vi "Convert to MessagePackT format byte.vi"(8 "error in (no error)":errorcluster, 11 "Object type":T1) -> (0 "error out":errorcluster, 3 "Byte":u8)   [LabVIEW 2020]
uses:
  MsgPack Object Types.ctl
  <vilib>/ErrorRing/Error Ring.xnode
  MessagePack.lvclass/MessagePack.ctl
  MessagePack.lvclass
  <vilib>/Utility/error.llb/Error Cluster From Error Code.vi
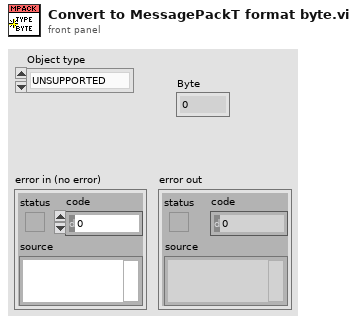
[diagram p1: front panel]
types:
  T1 = typedef "MessagePack.lvlib/MessagePack.lvclass/MsgPack Object Types.ctl" = enum16{"UNSUPPORTED", "POSINT", "NEGINT", "FIXMAP", "FIXARRAY", "FIXSTR", "NIL", "FALSE", "TRUE", "BIN8", "BIN16", "BIN32", "EXT8", "EXT16", "EXT32", "FLOAT32", "FLOAT64", "UINT8", "UINT16", "UINT32", "UINT64", "INT8", "INT16", "INT32", "INT64", "FIXEXT1", "FIXEXT2", "FIXEXT4", "FIXEXT8", "FIXEXT16", "STR8", "STR16", "STR32", "ARRAY16", "ARRAY32", "MAP16", "MAP32"}
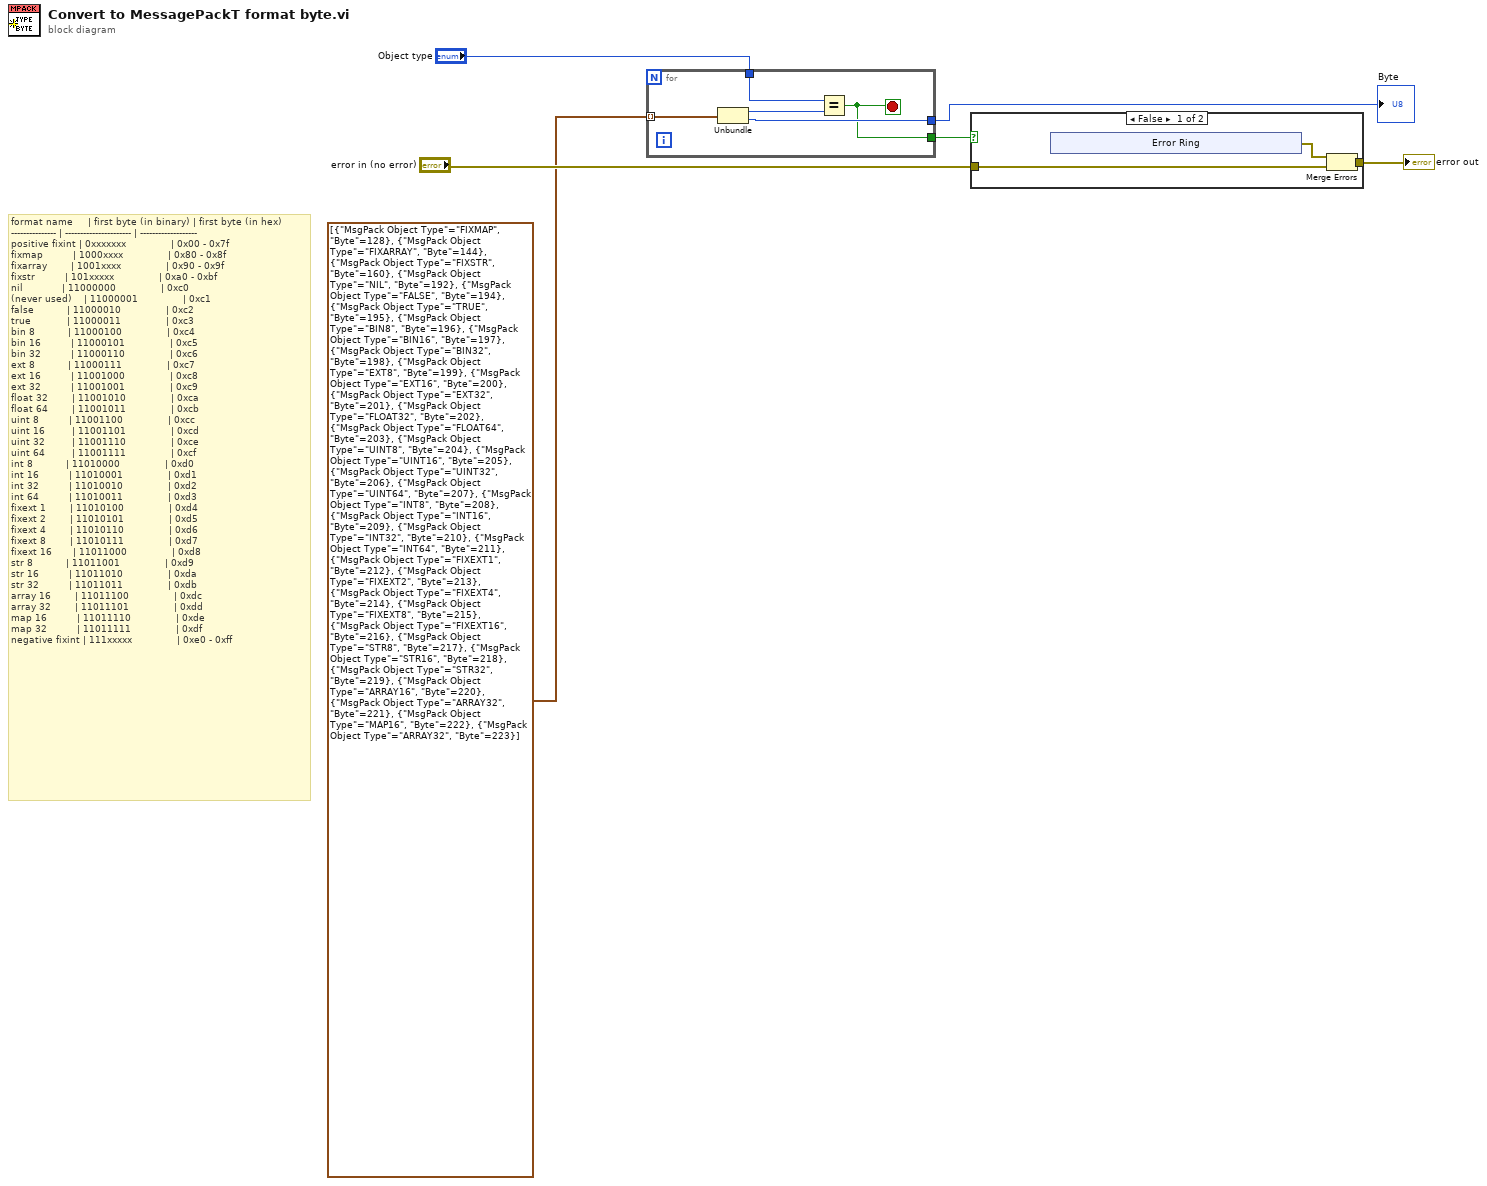
[diagram p0: block diagram]
diagram:
  # "format name     | first byte (in binary) | first byte (in hex)\n--------------- | ---------------------- | -------------------\npositive fixint | 0xxxxxxx               | 0x00 - 0x7f\nfixmap          | 1000xxxx               | 0x80 - 0x8f\nfixarray        | 1001xxxx               | 0x90 - 0x9f\nfixstr          | 101xxxxx               | 0xa0 - 0xbf\nnil             | 11000000               | 0xc0\n(never used)    | 11000001               | 0xc1\nfalse           | 11000010               | 0xc2\ntrue            | 11000011               | 0xc3\nbin 8           | 11000100               | 0xc4\nbin 16          | 11000101               | 0xc5\nbin 32          | 11000110               | 0xc6\next 8           | 11000111               | 0xc7\next 16          | 11001000               | 0xc8\next 32          | 11001001               | 0xc9\nfloat 32        | 11001010               | 0xca\nfloat 64        | 11001011               | 0xcb\nuint 8          | 11001100               | 0xcc\nuint 16         | 11001101               | 0xcd\nuint 32         | 11001110               | 0xce\nuint 64         | 11001111               | 0xcf\nint 8           | 11010000               | 0xd0\nint 16          | 11010001               | 0xd1\nint 32          | 11010010               | 0xd2\nint 64          | 11010011               | 0xd3\nfixext 1        | 11010100               | 0xd4\nfixext 2        | 11010101               | 0xd5\nfixext 4        | 11010110               | 0xd6\nfixext 8        | 11010111               | 0xd7\nfixext 16       | 11011000               | 0xd8\nstr 8           | 11011001               | 0xd9\nstr 16          | 11011010               | 0xda\nstr 32          | 11011011               | 0xdb\narray 16        | 11011100               | 0xdc\narray 32        | 11011101               | 0xdd\nmap 16          | 11011110               | 0xde\nmap 32          | 11011111               | 0xdf\nnegative fixint | 111xxxxx               | 0xe0 - 0xff"
  n1 = for {
    tunnel: cluster{"MsgPack Object Type":T1, "Byte":u8}[] [{"MsgPack Object Type"=enum."FIXMAP", "Byte"=128}, {"MsgPack Object Type"=enum."FIXARRAY", "Byte"=144}, {"MsgPack Object Type"=enum."FIXSTR", "Byte"=160}, {"MsgPack Object Type"=enum."NIL", "Byte"=192}, {"MsgPack Object Type"=enum."FALSE", "Byte"=194}, {"MsgPack Object Type"=enum."TRUE", "Byte"=195}, {"MsgPack Object Type"=enum."BIN8", "Byte"=196}, {"MsgPack Object Type"=enum."BIN16", "Byte"=197}, {"MsgPack Object Type"=enum."BIN32", "Byte"=198}, {"MsgPack Object Type"=enum."EXT8", "Byte"=199}, {"MsgPack Object Type"=enum."EXT16", "Byte"=200}, {"MsgPack Object Type"=enum."EXT32", "Byte"=201}, {"MsgPack Object Type"=enum."FLOAT32", "Byte"=202}, {"MsgPack Object Type"=enum."FLOAT64", "Byte"=203}, {"MsgPack Object Type"=enum."UINT8", "Byte"=204}, {"MsgPack Object Type"=enum."UINT16", "Byte"=205}, {"MsgPack Object Type"=enum."UINT32", "Byte"=206}, {"MsgPack Object Type"=enum."UINT64", "Byte"=207}, {"MsgPack Object Type"=enum."INT8", "Byte"=208}, {"MsgPack Object Type"=enum."INT16", "Byte"=209}, {"MsgPack Object Type"=enum."INT32", "Byte"=210}, {"MsgPack Object Type"=enum."INT64", "Byte"=211}, {"MsgPack Object Type"=enum."FIXEXT1", "Byte"=212}, {"MsgPack Object Type"=enum."FIXEXT2", "Byte"=213}, {"MsgPack Object Type"=enum."FIXEXT4", "Byte"=214}, {"MsgPack Object Type"=enum."FIXEXT8", "Byte"=215}, {"MsgPack Object Type"=enum."FIXEXT16", "Byte"=216}, {"MsgPack Object Type"=enum."STR8", "Byte"=217}, {"MsgPack Object Type"=enum."STR16", "Byte"=218}, {"MsgPack Object Type"=enum."STR32", "Byte"=219}, {"MsgPack Object Type"=enum."ARRAY16", "Byte"=220}, {"MsgPack Object Type"=enum."ARRAY32", "Byte"=221}, {"MsgPack Object Type"=enum."MAP16", "Byte"=222}, {"MsgPack Object Type"=enum."ARRAY32", "Byte"=223}] ("Enum") -> [w11] mode=indexing
    tunnel: "Object type" -> [w9]
    tunnel: [w8] -> w1
    tunnel: [w7] -> w2
    stop <- w7 stop-if-true
    n2 = Unbundle(w11) -> ("MsgPack Object Type"=w10:T1, "Byte"=w8:u8)
    n3 = Equal?(x=w9, y=w10) -> (x = y?=w7:bool)
  }
  "Byte" <- w1
  n4 = case shown="False" w2 {
    tunnel: "error in (no error)" -> [w13 w19]
    tunnel: [w12 w19] -> w5
    frame False {
      n5 = xnode "Error Ring"() -> ("error out"=w14:errorcluster)
      n6 = Merge Errors(w14, w13) -> (w12:errorcluster)
    }
    frame True {
    }
  }
  "error out" <- w5
